vi "IviDmm - Single Point Measurement.vi"() -> ()   [LabVIEW 2016, in "IVI_DMM.lvlib"]
doc: "This VI shows how to use the IviDmm class VIs to read a measurement. Notice the order of the IviDmm component VIs in the block diagram. The first IviDmm VI is the IviDmm Initialize.vi, which provides a handle to the instrument. The last IviDmm VI in a sequence must be IviDmm close.vi.\n\nIVI CLASS COMPLIANCE REQUIRED:\nThis VI requires that the specific driver adhere to the Base Capability Group of the IviDmm class."
uses:
  IVI_DMM.lvlib
panel:
  out "while":i32
  out "For":i32
  in  "stop":bool
  out "Readings":dbl[](array[numeric]) format="%.7p"
  in  "IVI Logical Names":refnum<k15>[](array[refnum])
  # "(c) 2000-2015 National Instruments.  All Rights Reserved."
  # "Overview: Instructs the instrument to read a measurement.\nRequirements: IVI Compliance Package, IviDmm-compliant specific driver  \nInstructions:\n1. Download and install an IVI specific driver from ni.com/idnet.\n2. Create and configure a logical name in the IVI Drivers category in Measurement & Automation Explorer (MAX).\n3. In the IVI Logical Name control below, select the logical name you configured in MAX.\n4. Review values in other controls and change if necessary. Refer to the specific driver help for appropriate settings.\n5. Run the VI."
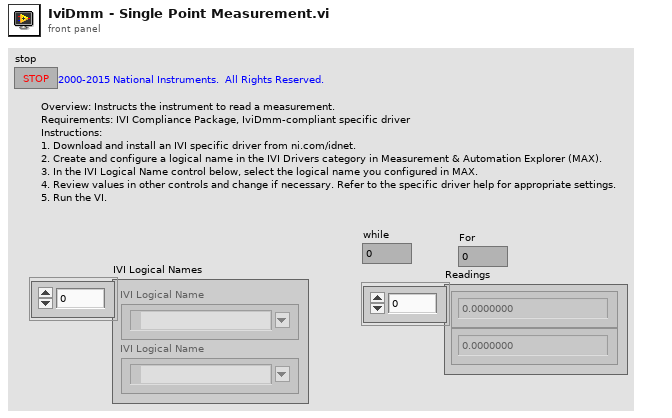
[diagram p1: front panel]
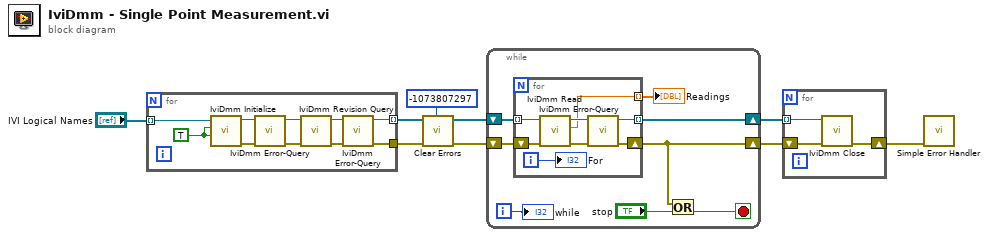
[diagram p0: block diagram]
diagram:
  n1 = for {
    tunnel: [w11] -> w5 mode=indexing
    tunnel: [w10] -> w4
    tunnel: "IVI Logical Names" -> [w17] mode=indexing
    w18 = TRUE ("reset device (true)")
    n2 = call <vilib>:"IviDmm Initialize.vi"("reset device (True)"=w18, "id query (True)"=w18, "logical name (\"SampleDmm\")"=w17) -> ("error out"=w12:errorcluster, "instrument handle out"=w16:refnum<k15>)  [unwired: 1 in, 6 out]
    n3 = call <vilib>:"IviDmm Error-Query.vi"("error in (no error)"=w12, "instrument handle"=w16) -> ("error out"=w13:errorcluster, "instrument handle out"=w14:refnum<k15>)  [unwired: 6 in, 2 out]
    n4 = call <vilib>:"IviDmm Revision Query.vi"("error in (no error)"=w13, "instrument handle"=w14) -> ("error out"=w9:errorcluster, "instrument handle out"=w15:refnum<k15>)  [unwired: 6 in, 2 out]
    n5 = call <vilib>:"IviDmm Error-Query.vi"("error in (no error)"=w9, "instrument handle"=w15) -> ("error out"=w10:errorcluster, "instrument handle out"=w11:refnum<k15>)  [unwired: 6 in, 2 out]
  }
  n6 = call <vilib>:"Clear Errors.vi"("error in (no error)"=w4, "specific error code to clear (0: all)"=-1073807297) -> ("error out"=w2:errorcluster)  [unwired: 4 in, 1 out]
  n7 = while {
    shift-right: [w26] -> w6
    shift-left: w5 -> [w25]
    shift-right: [w20] -> w8
    shift-left: w2 -> [w24]
    i -> [w19]
    stop <- w21 stop-if-true
    n8 = for {
      tunnel: [w31] -> w23 mode=indexing
      shift-right: [w29] -> w20
      shift-left: w24 -> [w32]
      tunnel: w25 -> [w33] mode=indexing
      tunnel: [w30] -> w26 mode=indexing
      i -> [w27]
      n9 = call <vilib>:"IviDmm Read.vi"("error in (no error)"=w32, "instrument handle"=w33) -> ("error out"=w28:errorcluster, "reading"=w31:dbl, "instrument handle out"=w34:refnum<k15>)  [unwired: 1 in, 6 out]
      n10 = call <vilib>:"IviDmm Error-Query.vi"("error in (no error)"=w28, "instrument handle"=w34) -> ("error out"=w29:errorcluster, "instrument handle out"=w30:refnum<k15>)  [unwired: 6 in, 2 out]
      "For" <- w27
    }
    "Readings" <- w23
    n11 = Or(x=w20, y="stop") -> (x .or. y?=w21:bool)
    "while" <- w19
  }
  n12 = for {
    tunnel: w6 -> [w35] mode=indexing
    shift-right: [w36] -> w7
    shift-left: w8 -> [w37]
    n13 = call <vilib>:"IviDmm Close.vi"("error in (no error)"=w37, "instrument handle"=w35) -> ("error out"=w36:errorcluster)  [unwired: 9 out]
  }
  n14 = call <vilib>:"Simple Error Handler.vi"("error in (no error)"=w7) -> ()  [unwired: 4 in, 5 out]
